vi "Radau5_Formula String Function.vi"(2 "data":variant, 3 "t":dbl, 4 "X'":dbl[](array[numeric]), 5 "X":dbl[](array[numeric])) -> (0 "error out":errorcluster, 1 "F(X,X',t)":dbl[](array[numeric]))   [LabVIEW 2017, in "NI_DAE.lvlib"]
uses:
  <vilib>/gmath/NI_DAE.lvlib
  <vilib>/gmath/NI_Gmath.lvlib
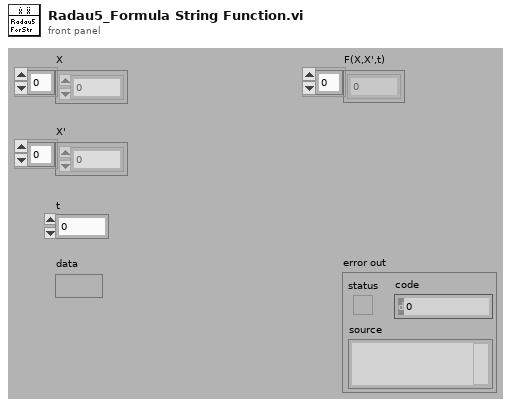
[diagram p1: front panel]
types:
  T1 = cluster{"F(X,X',t)":string[], "X":string[], "X'":string[], "time":string}
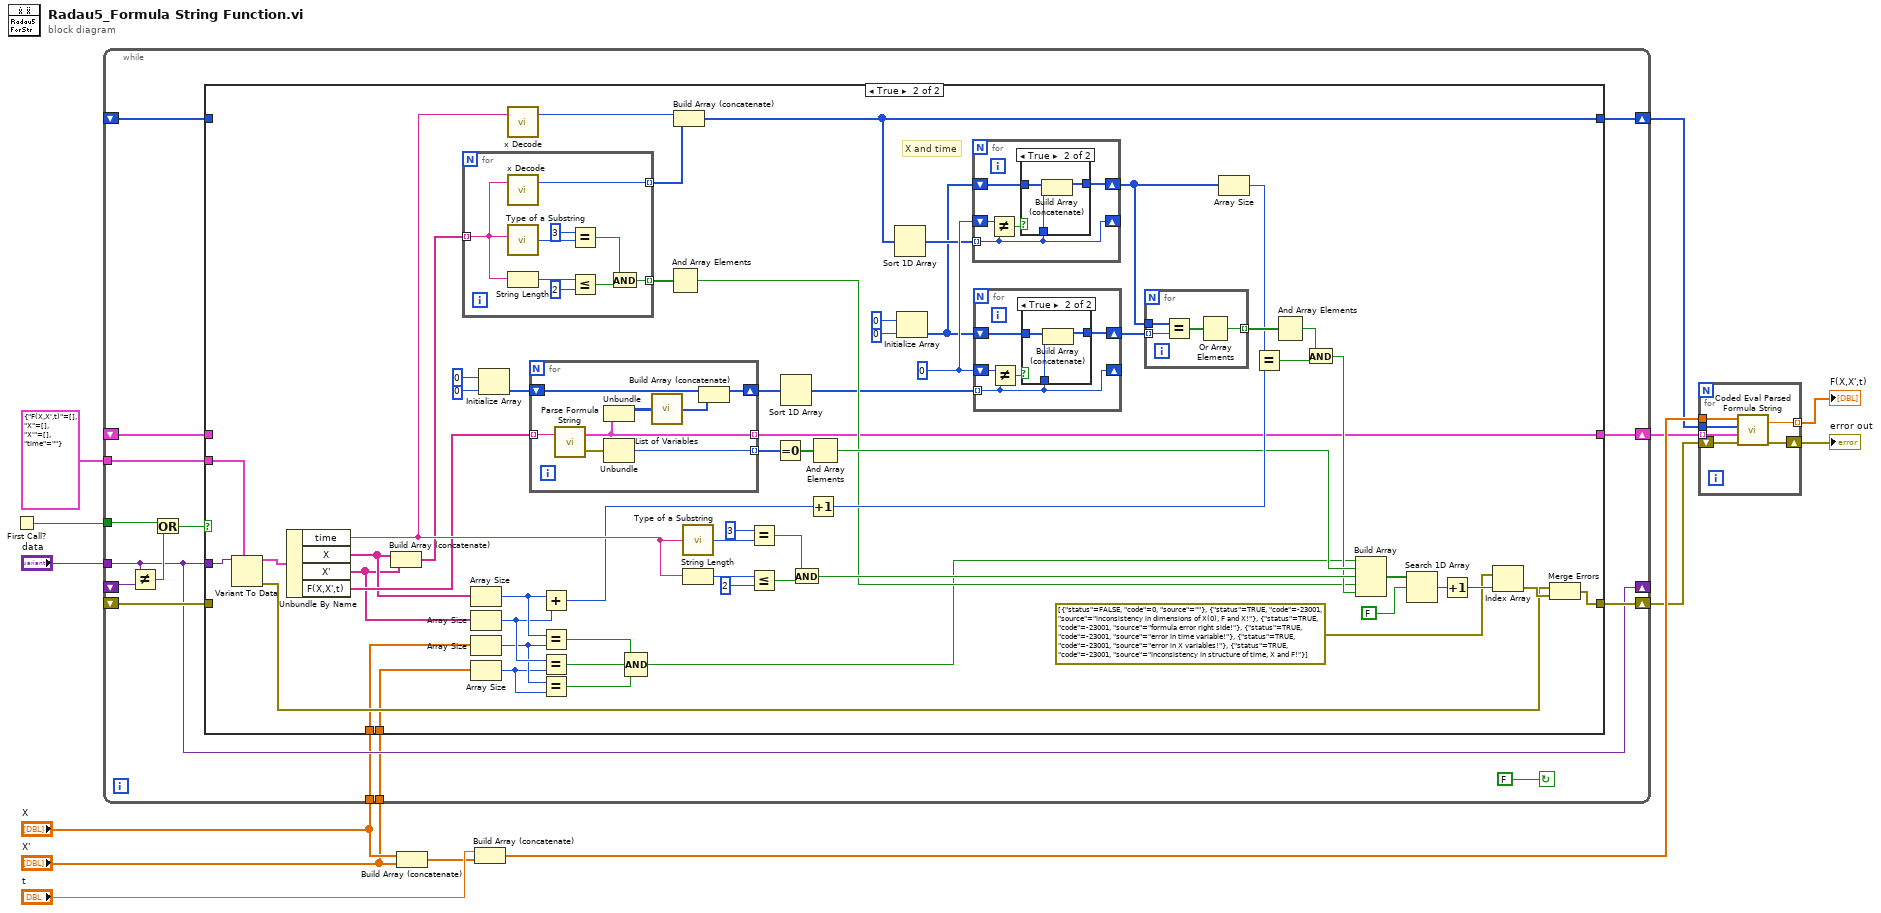
[diagram p0: block diagram]
diagram:
  n1 = First Call?() -> (First Call?: T/F=w13:bool)
  n2 = while {
    tunnel: w13 -> [w19]
    tunnel: "data" -> [w17]
    shift-right: [w25] -> w11
    shift-left: _ -> [w24]
    shift-right: [w27] -> w9
    shift-left: _ -> [w26]
    shift-right: [w23] -> w10
    shift-left: _ -> [w22]
    shift-right: [w17] -> _
    shift-left: _ -> [w21]
    tunnel: T1 {"F(X,X',t)"=[], "X"=[], "X'"=[], "time"=""} ("DAE F(X,X',t)") -> [w16]
    tunnel: "X" -> [w15]
    tunnel: "X'" -> [w14]
    stop <- FALSE continue-if-true
    n3 = Not Equal?(x=w17, y=w21) -> (x != y?=w20:bool)
    n4 = Or(x=w19, y=w20) -> (x .or. y?=w18:bool)
    n5 = case shown="True" w18 {
      tunnel: w17 -> [_ w92]
      tunnel: [w31 w64] -> w27
      tunnel: w26 -> [w31 _]
      tunnel: [w30 w52] -> w25
      tunnel: w24 -> [w30 _]
      tunnel: [w29 w60] -> w23
      tunnel: w22 -> [w29 _]
      tunnel: w16 -> [_ w48]
      tunnel: w15 -> [_ w42]
      tunnel: w14 -> [_ w41]
      frame False {
      }
      frame True {
        w57 = 0
        # "X and time"
        n6 = Variant To Data(type=w48, Variant=w92) -> (data=w76:T1, error out=w65:errorcluster)  [unwired: 1 in]
        n7 = Unbundle By Name(w76) -> ("time"=w63:string, "X"=w44:string[], "X'"=w43:string[], "F(X,X',t)"=w47:string[])
        n8 = Build Array (concatenate)(w44, w43) -> (w46:string[])
        n9 = for {
          tunnel: w46 -> [w116] mode=indexing
          tunnel: [w117] -> w85 mode=indexing
          tunnel: [w115] -> w62 mode=indexing
          n10 = call <vilib>:"x Decode.vi"("x string"=w116) -> ("number"=w115:i32)  [unwired: 1 in, 1 out]
          n11 = call <vilib>:"Type of a Substring.VI"("item"=w116) -> ("type"=w120:i32)
          n12 = String Length(string=w116) -> (length=w118:i32)
          n13 = Equal?(x=3, y=w120) -> (x = y?=w123:bool)
          n14 = Less Or Equal?(x=w118, y=2) -> (x <= y?=w122:bool)
          n15 = And(x=w123, y=w122) -> (x .and. y?=w117:bool)
        }
        n16 = Array Size(array=w44) -> (size(s)=w39:i32)
        n17 = Array Size(array=w43) -> (size(s)=w38:i32)
        n18 = Array Size(array=w42) -> (size(s)=w37:i32)
        n19 = Array Size(array=w41) -> (size(s)=w36:i32)
        n20 = Initialize Array(0, 0) -> (w88:i32[])
        n21 = call <vilib>:"x Decode.vi"("x string"=w63) -> ("number"=w61:i32)  [unwired: 1 in, 1 out]
        n22 = for {
          tunnel: [w126] -> w78 mode=indexing
          tunnel: w47 -> [w131] mode=indexing
          shift-right: [w129] -> w89
          shift-left: w88 -> [w130]
          tunnel: [w124] -> w60 mode=indexing
          n23 = call <vilib>:"Parse Formula String.vi"("formula"=w131) -> ("error out"=w127:errorcluster, "Parsed Formula"=w124:cluster{"Table":i32[][], "Y Values":dbl[]})  [unwired: 1 in]
          n24 = Unbundle(w124) -> ("Table"=w125:i32[][])  [unwired: 1 out]
          n25 = Unbundle(w127) -> ("code"=w126:i32)  [unwired: 2 out]
          n26 = call <vilib>:"List of Variables.vi"("Table"=w125) -> ("List of variables"=w128:i32[])
          n27 = Build Array (concatenate)(w130, w128) -> (w129:i32[])
        }
        n28 = Add(x=w39, y=w38) -> (x+y=w40:i32)
        n29 = Equal?(x=w39, y=w37) -> (x = y?=w35:bool)
        n30 = Equal?(x=w38, y=w36) -> (x = y?=w34:bool)
        n31 = Equal?(x=w37, y=w36) -> (x = y?=w33:bool)
        n32 = Compound Arithmetic op=AND(w35, w34, w33) -> (w32:bool)
        n33 = And Array Elements(Boolean array=w85) -> (logical AND=w72:bool)
        n34 = Build Array (concatenate)(w61, w62) -> (w52:i32[])
        n35 = call <vilib>:"Type of a Substring.VI"("item"=w63) -> ("type"=w81:i32)
        n36 = String Length(string=w63) -> (length=w79:i32)
        n37 = Equal?(x=3, y=w81) -> (x = y?=w84:bool)
        n38 = Less Or Equal?(x=w79, y=2) -> (x <= y?=w83:bool)
        n39 = Equal To 0?(x=w78) -> (x = 0?=w77:bool[])
        n40 = Sort 1D Array(array=w89) -> (sorted array=w51:i32[])
        n41 = And(x=w84, y=w83) -> (x .and. y?=w74:bool)
        n42 = Increment(x=w40) -> (x+1=w90:i32)
        n43 = And Array Elements(Boolean array=w77) -> (logical AND=w75:bool)
        n44 = Sort 1D Array(array=w52) -> (sorted array=w56:i32[])
        n45 = Initialize Array(0, 0) -> (w45:i32[])
        n46 = for {
          shift-right: [w103] -> w54
          shift-left: w45 -> [w104]
          shift-right: [w102] -> _
          shift-left: w57 -> [w106]
          tunnel: w56 -> [w102] mode=indexing
          n47 = Not Equal?(x=w106, y=w102) -> (x != y?=w105:bool)
          n48 = case shown="True" w105 {
            tunnel: w104 -> [w107 w110]
            tunnel: [w107 w109] -> w103
            tunnel: w102 -> [_ w108]
            frame False {
            }
            frame True {
              n49 = Build Array (concatenate)(w110, w108) -> (w109:i32[])
            }
          }
        }
        n50 = for {
          shift-right: [w94] -> w55
          shift-left: w45 -> [w95]
          shift-right: [w93] -> _
          shift-left: w57 -> [w97]
          tunnel: w51 -> [w93] mode=indexing
          n51 = Not Equal?(x=w97, y=w93) -> (x != y?=w96:bool)
          n52 = case shown="True" w96 {
            tunnel: w95 -> [w98 w101]
            tunnel: [w98 w100] -> w94
            tunnel: w93 -> [_ w99]
            frame False {
            }
            frame True {
              n53 = Build Array (concatenate)(w101, w99) -> (w100:i32[])
            }
          }
        }
        n54 = for {
          tunnel: w55 -> [w114] mode=indexing
          tunnel: w54 -> [w113]
          tunnel: [w111] -> w53 mode=indexing
          n55 = Equal?(x=w113, y=w114) -> (x = y?=w112:bool[])
          n56 = Or Array Elements(Boolean array=w112) -> (logical OR=w111:bool)
        }
        n57 = Array Size(array=w54) -> (size(s)=w50:i32)
        n58 = Equal?(x=w50, y=w90) -> (x = y?=w91:bool)
        n59 = And Array Elements(Boolean array=w53) -> (logical AND=w49:bool)
        n60 = And(x=w49, y=w91) -> (x .and. y?=w73:bool)
        n61 = Build Array(w32, w75, w74, w72, w73) -> (w71:bool[])
        n62 = Search 1D Array(1D array=w71, element=FALSE) -> (index of element=w69:i32)  [unwired: 1 in]
        n63 = Increment(x=w69) -> (x+1=w68:i32)
        n64 = Index Array(array=errorcluster[] [{"status"=FALSE, "code"=0, "source"=""}, {"status"=TRUE, "code"=-23001, "source"="inconsistency in dimensions of X(0), F and X!"}, {"status"=TRUE, "code"=-23001, "source"="formula error right side!"}, {"status"=TRUE, "code"=-23001, "source"="error in time variable!"}, {"status"=TRUE, "code"=-23001, "source"="error in X variables!"}, {"status"=TRUE, "code"=-23001, "source"="inconsistency in structure of time, X and F!"}], index=w68) -> (element=w67:errorcluster)
        n65 = Merge Errors(w65, w67) -> (w64:errorcluster)
      }
    }
  }
  n66 = Build Array (concatenate)("X", "X'") -> (w4:dbl[])
  n67 = Build Array (concatenate)("t", w4) -> (w12:dbl[])
  n68 = for {
    tunnel: w11 -> [w135]
    tunnel: w12 -> [w136]
    tunnel: [w137] -> w8 mode=indexing
    shift-right: [w133] -> w7
    shift-left: w9 -> [w134]
    tunnel: w10 -> [w132] mode=indexing
    n69 = call <vilib>:"Coded Eval Parsed Formula String.vi"("error in (no error)"=w134, "Parsed Formula"=w132, "Variables"=w135, "X Values"=w136) -> ("error out"=w133:errorcluster, "y value"=w137:dbl)
  }
  "F(X,X',t)" <- w8
  "error out" <- w7
